vi "FRIC_navX_Internal_Serial_GenerateCommand.vi"(11 "Serial Process Loop TypeDef (in)":T1={"State Array"=[enum."INI", enum."Open"], "error"={"status"=FALSE, "code"=0, "source"=""}, "FPGA Cluster"={"Last Valid FPGA Time"=0.0, "Error Count"=0, "Initialized"=FALSE}, "Device Info"={"Interface"={"Protocol"=enum."SERIAL", "Update Rate (4Hz-200Hz)"=4, "navX Open TypeDef"=variant}, "Notify Packet"=refnum, "Loop VI Refnum"=refnum, "Ready to Close Occurrence Refnum"=refnum, "Name"=""}, "I2CDevRef"={"DevStatus"={"status"=FALSE, "code"=0, "source"=""}, "Device Address"=0, "Handle"=0, "I2C Bus"=enum."Invalid"}, "Registry"=[], "Command Array"=[214, 32], "Connected?"=FALSE, "navX Device Memory Size"=85, "notification"={"navX Action"=enum."None", "Data"=variant, "Stream Type"=enum."YRPH", "Device Number"=enum."Dev0"}, "Memory Size Set"=FALSE, "SPIDevRef"={"DevStatus"={"status"=FALSE, "code"=0, "source"=""}, "Handle"=0, "SPI Bus"=enum."SPI On-Board, CS0"}, "navX Serial Open"={"Stream Type"=enum."YRPH", "Serial Port"=enum."Onboard RS-232"}, "SerialPortRef"={"DevStatus"={"status"=FALSE, "code"=0, "source"=""}, "Serial Port Name"=""}, "Serial Read Buffer"="", "Serial Write Buffer"=[], "Device Number"=enum."Dev0", "navX SPI Open"={"SPI Bus"=enum."SPI MXP", "Clock Rate (Hz)"=500000.0}, "Loop dt"=0, "current time"=timestamp(0 s since 1904-01-01), "Loop Time"=0} {"navX Device Memory Size" format="%x"; "Command Array" items=["UNDEFINED"=0, "NAVX_INTEGRATION_CTL_RESET_VEL_X"=1, "NAVX_INTEGRATION_CTL_RESET_VEL_Y"=2, "NAVX_INTEGRATION_CTL_RESET_VEL_Z"=4, "NAVX_INTEGRATION_CTL_RESET_DISP_X"=8, "NAVX_INTEGRATION_CTL_RESET_DISP_Y"=16, "NAVX_INTEGRATION_CTL_RESET_DISP_Z"=32, "NAVX_INTEGRATION_CTL_RESET_YAW"=128]; "I2CDevRef"."Device Address" format="%.0x"; "Device Info"."Interface"."Update Rate (4Hz-200Hz)" min=4 max=200 step=1}) -> (3 "Serial Process Loop TypeDef (out)":T1={"State Array"=[enum."INI", enum."Open"], "error"={"status"=FALSE, "code"=0, "source"=""}, "FPGA Cluster"={"Last Valid FPGA Time"=0.0, "Error Count"=0, "Initialized"=FALSE}, "Device Info"={"Interface"={"Protocol"=enum."SERIAL", "Update Rate (4Hz-200Hz)"=4, "navX Open TypeDef"=variant}, "Notify Packet"=refnum, "Loop VI Refnum"=refnum, "Ready to Close Occurrence Refnum"=refnum, "Name"=""}, "I2CDevRef"={"DevStatus"={"status"=FALSE, "code"=0, "source"=""}, "Device Address"=0, "Handle"=0, "I2C Bus"=enum."Invalid"}, "Registry"=[], "Command Array"=[], "Connected?"=FALSE, "navX Device Memory Size"=85, "notification"={"navX Action"=enum."None", "Data"=variant, "Stream Type"=enum."YRPH", "Device Number"=enum."Dev0"}, "Memory Size Set"=FALSE, "SPIDevRef"={"DevStatus"={"status"=FALSE, "code"=0, "source"=""}, "Handle"=0, "SPI Bus"=enum."SPI On-Board, CS0"}, "navX Serial Open"={"Stream Type"=enum."YRPH", "Serial Port"=enum."Onboard RS-232"}, "SerialPortRef"={"DevStatus"={"status"=FALSE, "code"=0, "source"=""}, "Serial Port Name"=""}, "Serial Read Buffer"="", "Serial Write Buffer"=[], "Device Number"=enum."Dev0", "navX SPI Open"={"SPI Bus"=enum."SPI MXP", "Clock Rate (Hz)"=500000.0}, "Loop dt"=0, "current time"=timestamp(0 s since 1904-01-01), "Loop Time"=0} {"navX Device Memory Size" format="%x"; "Command Array" items=["UNDEFINED"=0, "NAVX_INTEGRATION_CTL_RESET_VEL_X"=1, "NAVX_INTEGRATION_CTL_RESET_VEL_Y"=2, "NAVX_INTEGRATION_CTL_RESET_VEL_Z"=4, "NAVX_INTEGRATION_CTL_RESET_DISP_X"=8, "NAVX_INTEGRATION_CTL_RESET_DISP_Y"=16, "NAVX_INTEGRATION_CTL_RESET_DISP_Z"=32, "NAVX_INTEGRATION_CTL_RESET_YAW"=128]; "I2CDevRef"."Device Address" format="%.0x"; "Device Info"."Interface"."Update Rate (4Hz-200Hz)" min=4 max=200 step=1})   [LabVIEW 2019]
uses:
  _TypeDefs/FRIC_navX_I2C Process Loop TypeDef.ctl
  _TypeDefs/FRIC_navX_ProcessingLoopStatesTypeDef_I2C.ctl
  _TypeDefs/Z900_navX_DeviceTypeDef.ctl
  _TypeDefs/Z900_navX_ProtocolTypeDef.ctl
  _TypeDefs/Z900_navX_NotifyPacketTypeDef.ctl
  _TypeDefs/Z900_navX_ActionTypeDef.ctl
  _TypeDefs/Z900_navX_SerialStreamTypeDef.ctl
  _TypeDefs/FRIC_navX_DeviceNumbersTypeDef.ctl
  <vilib>/Rock Robotics/SystemInterfaces/i2clib/i2c_bus.ctl
  _TypeDefs/Z900_navX_IntegrationControlRegisters.ctl
  <vilib>/Rock Robotics/WPI/SPI/WPI_SPIDevRef.ctl
  <vilib>/Rock Robotics/SystemInterfaces/spilib/spi_bus.ctl
  <vilib>/Rock Robotics/WPI/SerialPort/WPI_SerialPort.ctl
  <vilib>/Rock Robotics/WPI/SerialPort/WPI_SerialPortRef.ctl
  _TypeDefs/Z900_navX_ZeroVectorTypeDef.ctl
panel:
  out "interleaved array":string[](array[string])
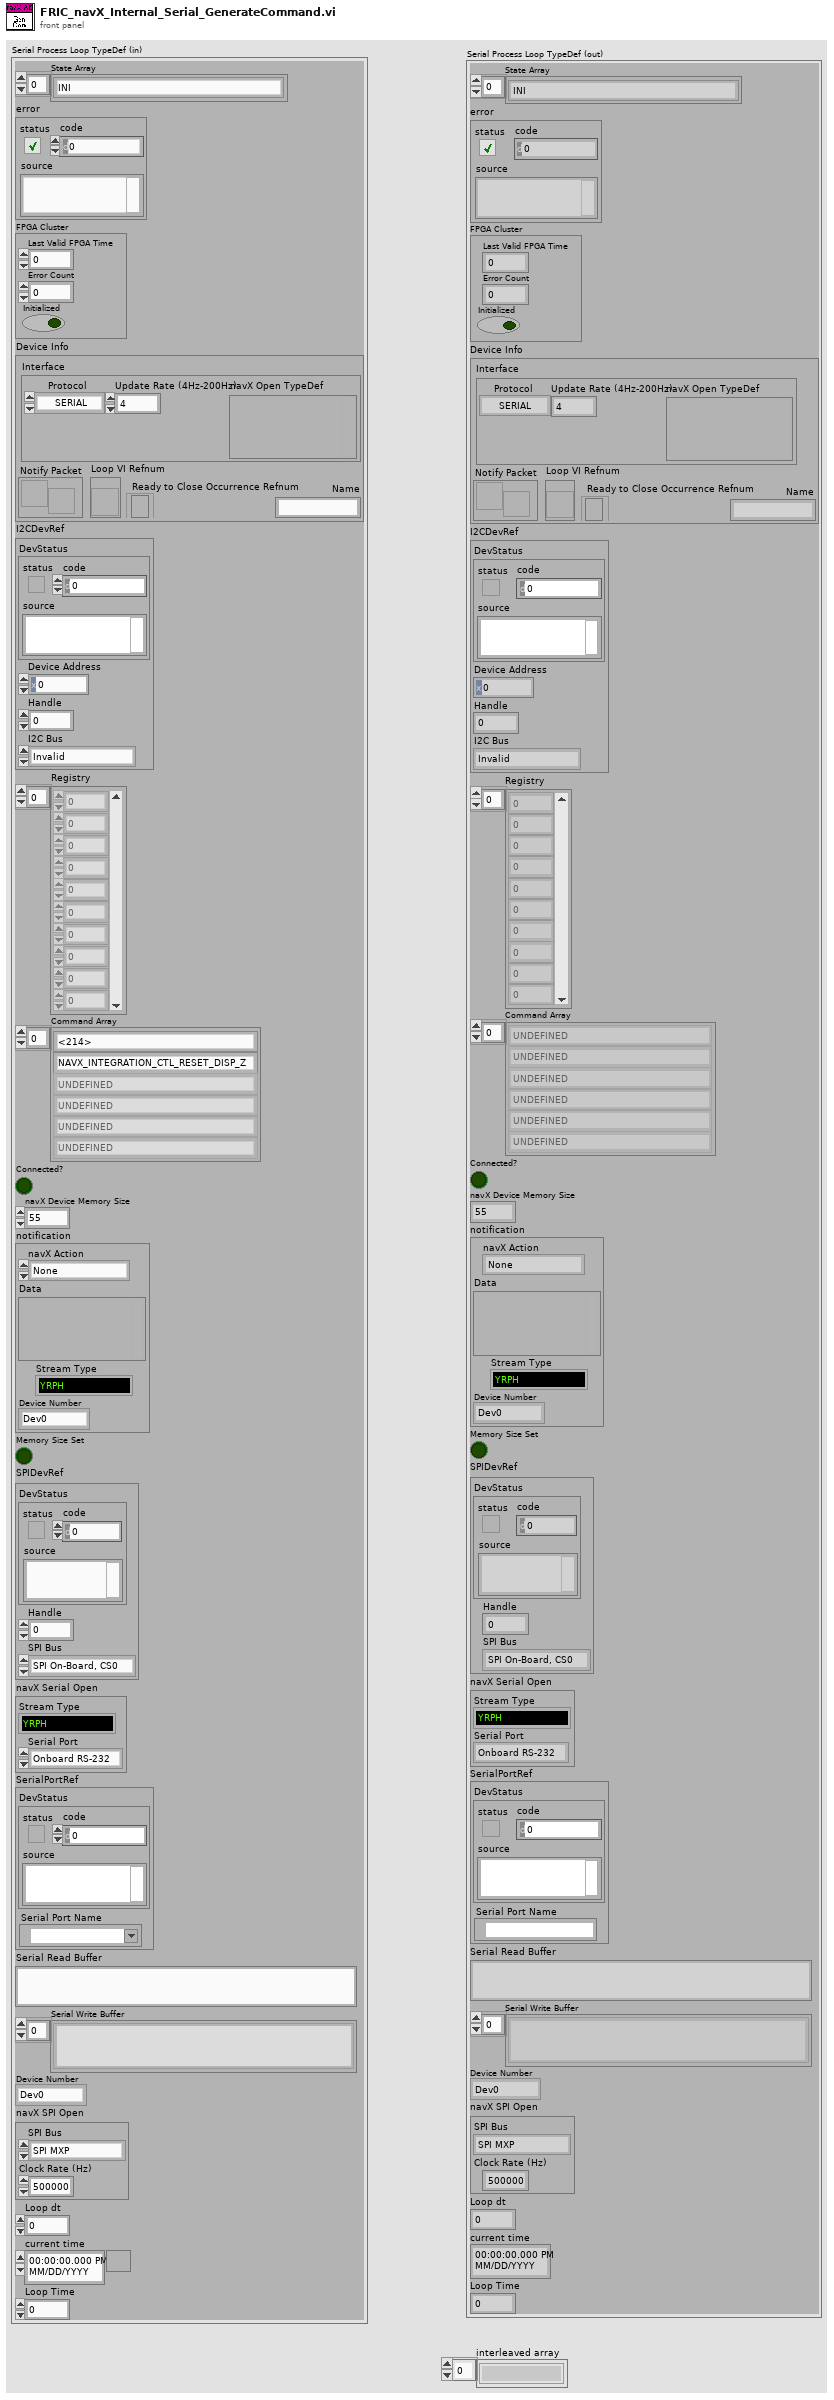
[diagram p1: front panel]
types:
  T1 = typedef "FRIC_navX_I2C Process Loop TypeDef.ctl" = cluster{"State Array":T2[], "error":errorcluster, "FPGA Cluster":cluster{"Last Valid FPGA Time":dbl, "Error Count":i32, "Initialized":bool}, "Device Info":T3, "I2CDevRef":cluster{"DevStatus":errorcluster, "Device Address":u8, "Handle":i32, "I2C Bus":T5}, "Registry":u8[], "Command Array":T6[], "Connected?":bool, "navX Device Memory Size":i32, "notification":T7, "Memory Size Set":bool, "SPIDevRef":T11, "navX Serial Open":cluster{"Stream Type":T9, "Serial Port":T13}, "SerialPortRef":T14, "Serial Read Buffer":string, "Serial Write Buffer":string[], "Device Number":T10, "navX SPI Open":cluster{"SPI Bus":T12, "Clock Rate (Hz)":dbl}, "Loop dt":i64, "current time":timestamp, "Loop Time":i64}
  T2 = typedef "FRIC_navX_ProcessingLoopStatesTypeDef_I2C.ctl" = enum16{"Process", "INI", "Check Packets Valid", "Close", "Clear VISA", "Generate Command", "Last Packet Valid", "Open", "Read", "Reset Serial", "Set Termination Char", "Update AE", "Wait", "Write", "Exit"}
  T3 = typedef "Z900_navX_DeviceTypeDef.ctl" = cluster{"Interface":cluster{"Protocol":T4, "Update Rate (4Hz-200Hz)":u8, "navX Open TypeDef":variant}, "Notify Packet":refnum<notifier>, "Loop VI Refnum":refnum<vi>, "Ready to Close Occurrence Refnum":refnum<k4>, "Name":string}
  T4 = typedef "Z900_navX_ProtocolTypeDef.ctl" = enum16{"SERIAL", "I2C", "SPI"}
  T5 = typedef "i2c_bus.ctl" = enum16{"I2C On-Board", "I2C MXP", "Invalid"}
  T6 = typedef "Z900_navX_IntegrationControlRegisters.ctl" = u8
  T7 = typedef "Z900_navX_NotifyPacketTypeDef.ctl" = cluster{"navX Action":T8, "Data":variant, "Stream Type":T9, "Device Number":T10}
  T8 = typedef "Z900_navX_ActionTypeDef.ctl" = enum16{"None", "Halt", "Normal Read", "Update Serial Protocol", "Update Rate Htz", "Zero-Yaw", "Zero-Displacement", "Zero-Velocity"}
  T9 = typedef "Z900_navX_SerialStreamTypeDef.ctl" = enum16{"YRPH", "Quaterinons", "Gyro/Raw", "AHRS", "AHRSAndPositioning", "AHRSAndPOSTime"}
  T10 = typedef "FRIC_navX_DeviceNumbersTypeDef.ctl" = enum16{"Dev0", "Dev1", "Dev2", "Dev3"}
  T11 = typedef "WPI_SPIDevRef.ctl" = cluster{"DevStatus":errorcluster, "Handle":i32, "SPI Bus":T12}
  T12 = typedef "spi_bus.ctl" = enum16{"SPI On-Board, CS0", "SPI On-Board, CS1", "SPI On-Board, CS2", "SPI On-Board, CS3", "SPI MXP", "Invalid"}
  T13 = typedef "WPI_SerialPort.ctl" = enum16{"Onboard RS-232", "MXP TTL", "USB 1", "USB 2"}
  T14 = typedef "WPI_SerialPortRef.ctl" = cluster{"DevStatus":errorcluster, "Serial Port Name":refnum<visa-resource-name>}
  T15 = typedef "Z900_navX_ZeroVectorTypeDef.ctl" = cluster{"X":bool, "Y":bool, "Z":bool}
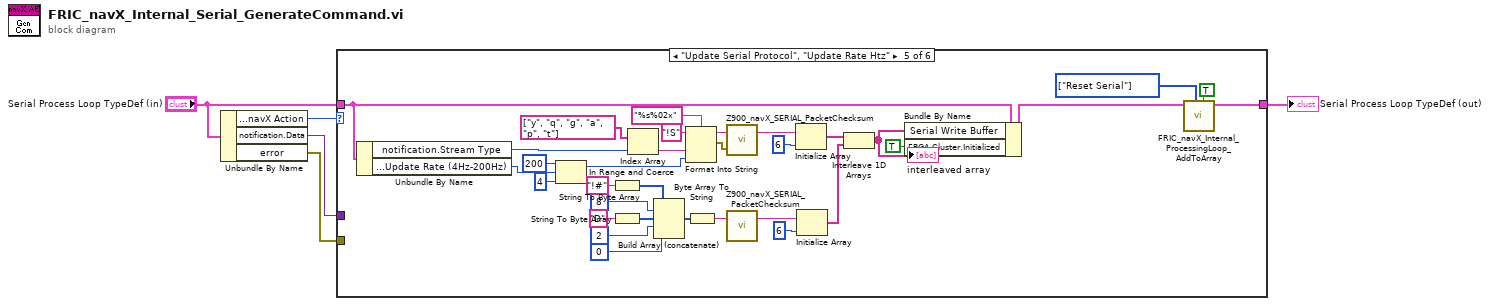
[diagram p0: block diagram]
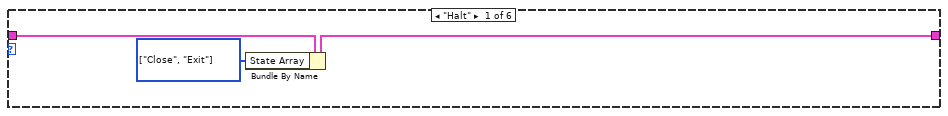
[diagram p2: hidden frame]
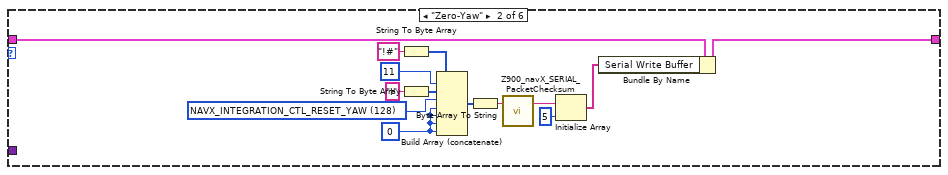
[diagram p3: hidden frame]
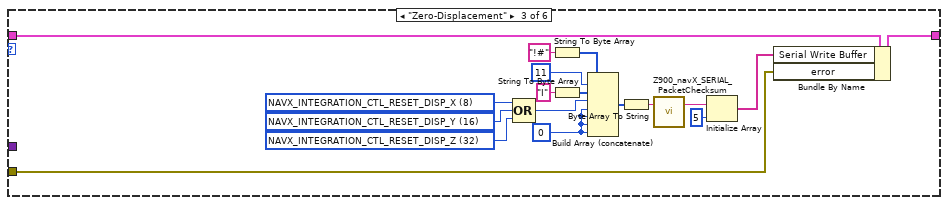
[diagram p4: hidden frame]
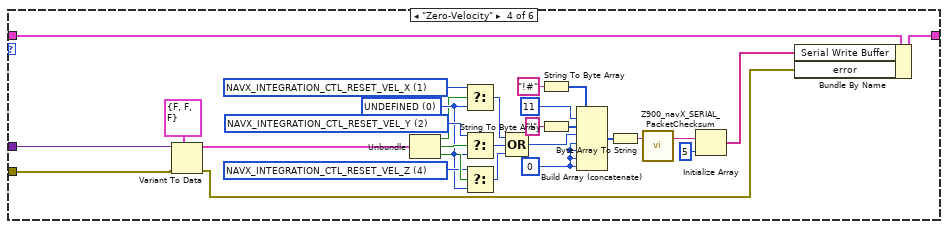
[diagram p5: hidden frame]
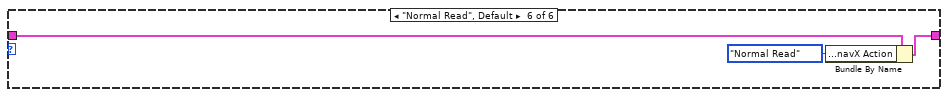
[diagram p6: hidden frame]
diagram:
  n1 = Unbundle By Name("Serial Process Loop TypeDef (in)") -> ("notification.navX Action"=w4:T8, "notification.Data"=w3:variant, "error"=w2:errorcluster)
  n2 = case shown="\"Update Serial Protocol\", \"Update Rate Htz\"" w4 {
    tunnel: "Serial Process Loop TypeDef (in)" -> [w8 w22 w39 w67 w102 w104]
    tunnel: [w7 w21 w40 w68 w78 w103] -> w1
    tunnel: w3 -> [_ _ _ w69 _ _]
    tunnel: w2 -> [_ _ w26 w66 _ _]
    frame "Halt" {
      w6 = T2[] [enum."Close", enum."Exit"] items=["Process", "INI", "Check Packets Valid", "Close", "Clear VISA", "Generate Command", "Last Packet Valid", "Open", "Read", "Reset Serial", "Set Termination Char", "Update AE", "Wait", "Write", "Exit"]
      n3 = Bundle By Name(cluster=w8, "State Array"=w6) -> (w7:T1)
    }
    frame "Zero-Yaw" {
      w18 = 0
      w12 = T6 128 items=["UNDEFINED"=0, "NAVX_INTEGRATION_CTL_RESET_VEL_X"=1, "NAVX_INTEGRATION_CTL_RESET_VEL_Y"=2, "NAVX_INTEGRATION_CTL_RESET_VEL_Z"=4, "NAVX_INTEGRATION_CTL_RESET_DISP_X"=8, "NAVX_INTEGRATION_CTL_RESET_DISP_Y"=16, "NAVX_INTEGRATION_CTL_RESET_DISP_Z"=32, "NAVX_INTEGRATION_CTL_RESET_YAW"=128] ("Integration Control Register")
      n4 = String To Byte Array(string="!#" ("initial string")) -> (unsigned byte array=w13:u8[])
      n5 = String To Byte Array(string="I" ("initial string")) -> (unsigned byte array=w15:u8[])
      n6 = Build Array (concatenate)(w13, 11, w15, w12, w18, w18, w18, w18) -> (w14:i32[])
      n7 = Byte Array To String(unsigned byte array=w14) -> (string=w10:string)
      n8 = call "Z900_navX_SERIAL_PacketChecksum.vi"("Packet"=w10) -> ("Terminated Packet"=w19:string)  [unwired: 1 in, 1 out]
      n9 = Initialize Array(w19, 5 ("dimension size")) -> (w9:string[])
      n10 = Bundle By Name(cluster=w22, "Serial Write Buffer"=w9) -> (w21:T1)
    }
    frame "Zero-Displacement" {
      w36 = 0
      w23 = T6 32 items=["UNDEFINED"=0, "NAVX_INTEGRATION_CTL_RESET_VEL_X"=1, "NAVX_INTEGRATION_CTL_RESET_VEL_Y"=2, "NAVX_INTEGRATION_CTL_RESET_VEL_Z"=4, "NAVX_INTEGRATION_CTL_RESET_DISP_X"=8, "NAVX_INTEGRATION_CTL_RESET_DISP_Y"=16, "NAVX_INTEGRATION_CTL_RESET_DISP_Z"=32, "NAVX_INTEGRATION_CTL_RESET_YAW"=128] ("Integration Control Register")
      w24 = T6 16 items=["UNDEFINED"=0, "NAVX_INTEGRATION_CTL_RESET_VEL_X"=1, "NAVX_INTEGRATION_CTL_RESET_VEL_Y"=2, "NAVX_INTEGRATION_CTL_RESET_VEL_Z"=4, "NAVX_INTEGRATION_CTL_RESET_DISP_X"=8, "NAVX_INTEGRATION_CTL_RESET_DISP_Y"=16, "NAVX_INTEGRATION_CTL_RESET_DISP_Z"=32, "NAVX_INTEGRATION_CTL_RESET_YAW"=128] ("Integration Control Register")
      w25 = T6 8 items=["UNDEFINED"=0, "NAVX_INTEGRATION_CTL_RESET_VEL_X"=1, "NAVX_INTEGRATION_CTL_RESET_VEL_Y"=2, "NAVX_INTEGRATION_CTL_RESET_VEL_Z"=4, "NAVX_INTEGRATION_CTL_RESET_DISP_X"=8, "NAVX_INTEGRATION_CTL_RESET_DISP_Y"=16, "NAVX_INTEGRATION_CTL_RESET_DISP_Z"=32, "NAVX_INTEGRATION_CTL_RESET_YAW"=128] ("Integration Control Register")
      n11 = Compound Arithmetic op=OR(w25, w24, w23) -> (w28:T6)
      n12 = String To Byte Array(string="!#" ("initial string")) -> (unsigned byte array=w31:u8[])
      n13 = String To Byte Array(string="I" ("initial string")) -> (unsigned byte array=w33:u8[])
      n14 = Build Array (concatenate)(w31, 11, w33, w28, w36, w36, w36, w36) -> (w32:i32[])
      n15 = Byte Array To String(unsigned byte array=w32) -> (string=w29:string)
      n16 = call "Z900_navX_SERIAL_PacketChecksum.vi"("Packet"=w29) -> ("Terminated Packet"=w37:string)  [unwired: 1 in, 1 out]
      n17 = Initialize Array(w37, 5 ("dimension size")) -> (w27:string[])
      n18 = Bundle By Name(cluster=w39, "Serial Write Buffer"=w27, "error"=w26) -> (w40:T1)
    }
    frame "Zero-Velocity" {
      w50 = 0
      w58 = T6 0 items=["UNDEFINED"=0, "NAVX_INTEGRATION_CTL_RESET_VEL_X"=1, "NAVX_INTEGRATION_CTL_RESET_VEL_Y"=2, "NAVX_INTEGRATION_CTL_RESET_VEL_Z"=4, "NAVX_INTEGRATION_CTL_RESET_DISP_X"=8, "NAVX_INTEGRATION_CTL_RESET_DISP_Y"=16, "NAVX_INTEGRATION_CTL_RESET_DISP_Z"=32, "NAVX_INTEGRATION_CTL_RESET_YAW"=128] ("f")
      w59 = T6 4 items=["UNDEFINED"=0, "NAVX_INTEGRATION_CTL_RESET_VEL_X"=1, "NAVX_INTEGRATION_CTL_RESET_VEL_Y"=2, "NAVX_INTEGRATION_CTL_RESET_VEL_Z"=4, "NAVX_INTEGRATION_CTL_RESET_DISP_X"=8, "NAVX_INTEGRATION_CTL_RESET_DISP_Y"=16, "NAVX_INTEGRATION_CTL_RESET_DISP_Z"=32, "NAVX_INTEGRATION_CTL_RESET_YAW"=128] ("Integration Control Register")
      w60 = T6 2 items=["UNDEFINED"=0, "NAVX_INTEGRATION_CTL_RESET_VEL_X"=1, "NAVX_INTEGRATION_CTL_RESET_VEL_Y"=2, "NAVX_INTEGRATION_CTL_RESET_VEL_Z"=4, "NAVX_INTEGRATION_CTL_RESET_DISP_X"=8, "NAVX_INTEGRATION_CTL_RESET_DISP_Y"=16, "NAVX_INTEGRATION_CTL_RESET_DISP_Z"=32, "NAVX_INTEGRATION_CTL_RESET_YAW"=128] ("Integration Control Register")
      w57 = T6 1 items=["UNDEFINED"=0, "NAVX_INTEGRATION_CTL_RESET_VEL_X"=1, "NAVX_INTEGRATION_CTL_RESET_VEL_Y"=2, "NAVX_INTEGRATION_CTL_RESET_VEL_Z"=4, "NAVX_INTEGRATION_CTL_RESET_DISP_X"=8, "NAVX_INTEGRATION_CTL_RESET_DISP_Y"=16, "NAVX_INTEGRATION_CTL_RESET_DISP_Z"=32, "NAVX_INTEGRATION_CTL_RESET_YAW"=128] ("Integration Control Register")
      n19 = Variant To Data(error in=w66, type=T15 {"X"=FALSE, "Y"=FALSE, "Z"=FALSE} ("Zero Vector"), Variant=w69) -> (data=w54:T15, error out=w53:errorcluster)
      n20 = Unbundle(w54) -> ("X"=w56:bool, "Y"=w61:bool, "Z"=w62:bool)
      n21 = Select(t=w57, s=w56, f=w58) -> (s? t:f=w63:T6)
      n22 = Select(t=w60, s=w61, f=w58) -> (s? t:f=w64:T6)
      n23 = Select(t=w59, s=w62, f=w58) -> (s? t:f=w65:T6)
      n24 = Compound Arithmetic op=OR(w63, w64, w65) -> (w42:T6)
      n25 = String To Byte Array(string="!#" ("initial string")) -> (unsigned byte array=w45:u8[])
      n26 = String To Byte Array(string="I" ("initial string")) -> (unsigned byte array=w47:u8[])
      n27 = Build Array (concatenate)(w45, 11, w47, w42, w50, w50, w50, w50) -> (w46:i32[])
      n28 = Byte Array To String(unsigned byte array=w46) -> (string=w43:string)
      n29 = call "Z900_navX_SERIAL_PacketChecksum.vi"("Packet"=w43) -> ("Terminated Packet"=w51:string)  [unwired: 1 in, 1 out]
      n30 = Initialize Array(w51, 5 ("dimension size")) -> (w41:string[])
      n31 = Bundle By Name(cluster=w67, "Serial Write Buffer"=w41, "error"=w53) -> (w68:T1)
    }
    frame "Update Serial Protocol", "Update Rate Htz" {
      w71 = T2[] [enum."Reset Serial"] items=["Process", "INI", "Check Packets Valid", "Close", "Clear VISA", "Generate Command", "Last Packet Valid", "Open", "Read", "Reset Serial", "Set Termination Char", "Update AE", "Wait", "Write", "Exit"] ("States Array")
      n32 = Unbundle By Name(w102) -> ("notification.Stream Type"=w97:T9, "Device Info.Interface.Update Rate (4Hz-200Hz)"=w74:u8)
      n33 = In Range and Coerce(upper limit=u8 200, x=w74, lower limit=u8 4) -> (coerced(x)=w73:u8)  [unwired: 1 out]
      n34 = String To Byte Array(string="!#" ("initial string")) -> (unsigned byte array=w90:u8[])
      n35 = String To Byte Array(string="D" ("initial string")) -> (unsigned byte array=w88:u8[])
      n36 = Index Array(array=string[] ["y", "q", "g", "a", "p", "t"], index=w97) -> (element=w98:string)
      n37 = Build Array (concatenate)(w90, 8, w88, 2, 0) -> (w85:i32[])
      n38 = Format Into String(format string="%s%02x", initial string="!S", w98, w73) -> (resulting string=w96:string, error out=w95:errorcluster)  [unwired: 1 in]
      n39 = Byte Array To String(unsigned byte array=w85) -> (string=w94:string)
      n40 = call "Z900_navX_SERIAL_PacketChecksum.vi"("error in (no error)"=w95, "Packet"=w96) -> ("Terminated Packet"=w82:string)  [unwired: 1 out]
      n41 = call "Z900_navX_SERIAL_PacketChecksum.vi"("Packet"=w94) -> ("Terminated Packet"=w84:string)  [unwired: 1 in, 1 out]
      n42 = Initialize Array(w82, 6 ("dimension size")) -> (w81:string[])
      n43 = Initialize Array(w84, 6 ("dimension size")) -> (w80:string[])
      n44 = Interleave 1D Arrays(w81, w80) -> (w79:string[])
      "interleaved array" <- w79
      n45 = Bundle By Name(cluster=w102, "Serial Write Buffer"=w79, "FPGA Cluster.Initialized"=TRUE) -> (w77:T1)
      n46 = call "FRIC_navX_Internal_ProcessingLoop_AddToArray.vi"("Add to beginning"=TRUE, "States Array"=w71, "I2C Process Loop TypeDef (in)"=w77) -> ("I2C Process Loop TypeDef (out)"=w78:T1)  [unwired: 8 in]
    }
    frame "Normal Read", Default {
      n47 = Bundle By Name(cluster=w104, "notification.navX Action"=Z900_navX_ActionTypeDef."Normal Read") -> (w103:T1)
    }
  }
  "Serial Process Loop TypeDef (out)" <- w1
